vi "Radau5_Get Delta Z.vi"(8 "Inverse Matrix JM_2":T1, 9 "Inverse Matrix JM_1":T2, 10 "Width":i32, 11 "Vector U in":dbl[](array[numeric])) -> (3 "Delta Z out":dbl[](array[numeric]))   [LabVIEW 2017, in "NI_DAE.lvlib"]
uses:
  <vilib>/gmath/NI_DAE.lvlib
  <vilib>/Analysis/Matrix/Datatypes/RealMatrix.ctl
  <vilib>/Analysis/Matrix/Datatypes/ComplexMatrix.ctl
  <vilib>/Analysis/7linalg.llb/Real Kronecker Product.vi
  <vilib>/Analysis/baseanly.llb/A x Vector (Optimized).vi
  <vilib>/Analysis/baseanly.llb/Complex A x Vector (Optimized).vi
  <vilib>/Analysis/7linalg.llb/Create Special Real Matrix.vi
  <vilib>/Analysis/Matrix/NI_Matrix.lvlib
  <vilib>/Analysis/NI_AALPro.lvlib
  <vilib>/Analysis/NI_AALBase.lvlib
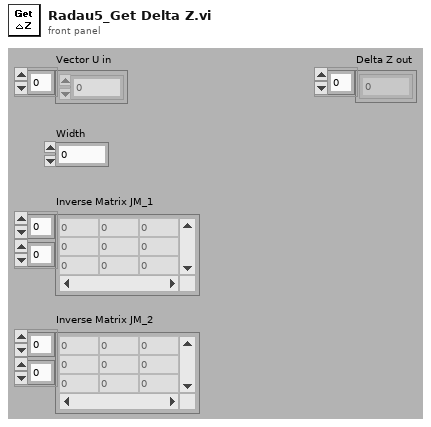
[diagram p1: front panel]
types:
  T1 = typedef "NI_Matrix.lvlib/ComplexMatrix.ctl" = cdb[][]
  T2 = typedef "NI_Matrix.lvlib/RealMatrix.ctl" = dbl[][]
  T3 = enum32{"Identity", "Diagonal", "Toepliz", "Vandermonde", "Companion"}
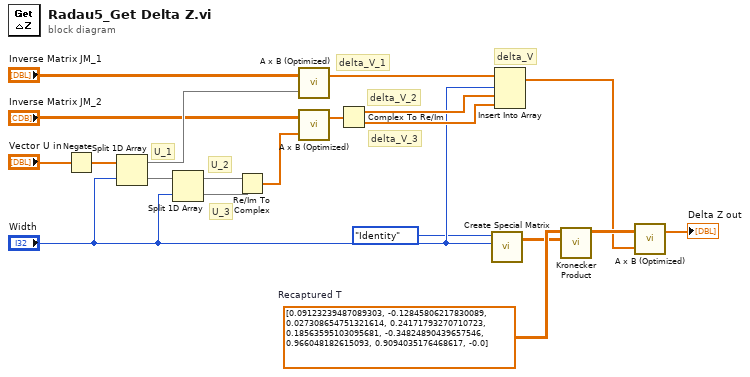
[diagram p0: block diagram]
diagram:
  w4 = T2 [[0.09123239487089303, -0.12845806217830089, 0.027308654751321614], [0.24171793270710723, 0.18563595103095681, -0.34824890439657546], [0.966048182615093, 0.9094035176468617, -0.0]]  # Recaptured T
  # "delta_V"
  # "delta_V_3"
  # "delta_V_2"
  # "delta_V_1"
  # "U_3"
  # "U_2"
  # "U_1"
  n1 = Negate(x="Vector U in") -> (-x=w11:dbl[])
  n2 = Split 1D Array(array=w11, index="Width") -> (first subarray=w15:dbl[], second subarray=w20:dbl[])
  n3 = Split 1D Array(array=w20, index="Width") -> (first subarray=w19:dbl[], second subarray=w18:dbl[])
  n4 = Re/Im To Complex(1:w18, 2:w19) -> (0:w13:cdb[])
  n5 = call-poly <vilib>:"A x B (Optimized).vi"("Vector"=w15, "A"="Inverse Matrix JM_1") -> ("A x Vector"=w10:dbl[])  [unwired: 1 out]
  n6 = call-poly <vilib>:"A x B (Optimized).vi"("Vector"=w13, "A"="Inverse Matrix JM_2") -> ("A x Vector"=w12:cdb[])  [unwired: 1 out]
  n7 = Complex To Re/Im(x + iy=w12) -> (x=w6:dbl[], y=w5:dbl[])
  n8 = call-poly <vilib>:"Create Special Matrix.vi"("matrix type"=T3."Identity", "matrix size"="Width") -> ("Special Matrix"=w1:T2)  [unwired: 3 in, 1 out]
  n9 = Insert Into Array(array=w10, index="Width", new element #1=w6, new element #2=w5) -> (w8:dbl[])
  n10 = call-poly <vilib>:"Kronecker Product.vi"("B"=w1, "A"=w4) -> ("Kronecker Product"=w9:T2)  [unwired: 9 out]
  n11 = call-poly <vilib>:"A x B (Optimized).vi"("Vector"=w8, "A"=w9) -> ("A x Vector"=→"Delta Z out":dbl[])  [unwired: 1 out]
